vi "aft_LMS_FPGA_Code_Generation.vi"(8 "read coefficient? (F)":bool, 9 "filter name":string, 10 "fixed-point LMS settings":T1, 11 "target item":refnum<vi>) -> (0 "error out":errorcluster, 2 "continue?":bool)   [LabVIEW 2017, in "NI_AdaptiveFilter.lvlib"]
uses:
  <vilib>/addons/Adaptive Filters/NI_AdaptiveFilter.lvlib
  <vilib>/addons/Adaptive Filters/Utilities/AFT Algorithm.ctl
  <vilib>/addons/Adaptive Filters/Utilities/AFT Errors.ctl
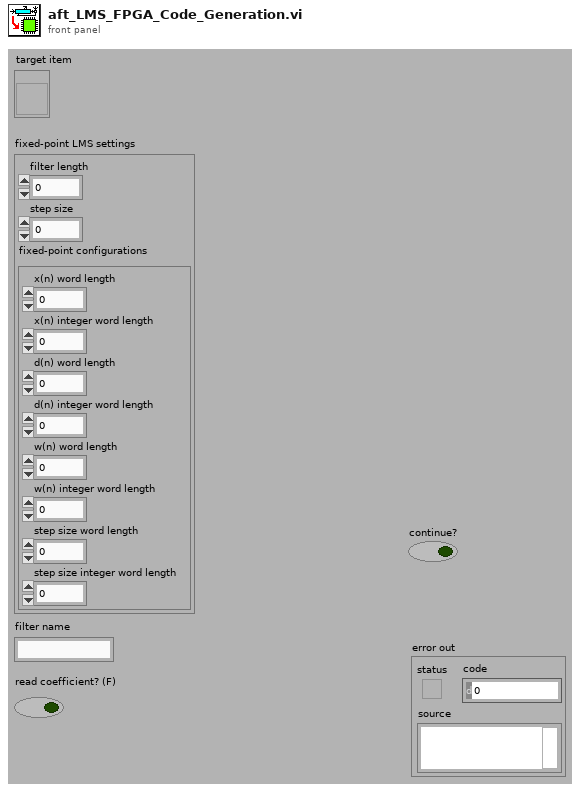
[diagram p1: front panel]
types:
  T1 = cluster{"filter length":i32, "step size":dbl, "fixed-point configurations":cluster{"x(n) word length":i32, "x(n) integer word length":i32, "d(n) word length":i32, "d(n) integer word length":i32, "w(n) word length":i32, "w(n) integer word length":i32, "step size word length":i32, "step size integer word length":i32}}
  T2 = typedef "NI_AdaptiveFilter.lvlib/AFT Errors.ctl" = i32
  T3 = typedef "NI_AdaptiveFilter.lvlib/AFT Algorithm.ctl" = u16
  T4 = cluster{"x(n) word length":i32, "x(n) integer word length":i32, "d(n) word length":i32, "d(n) integer word length":i32, "w(n) word length":i32, "w(n) integer word length":i32, "step size word length":i32, "step size integer word length":i32}
  T5 = cluster{"algorithm":T3, "filter length":i32, "step size":dbl, "fixed-point configurations":cluster{"x(n) word length":i32, "x(n) integer word length":i32, "d(n) word length":i32, "d(n) integer word length":i32, "w(n) word length":i32, "w(n) integer word length":i32, "step size word length":i32, "step size integer word length":i32}}
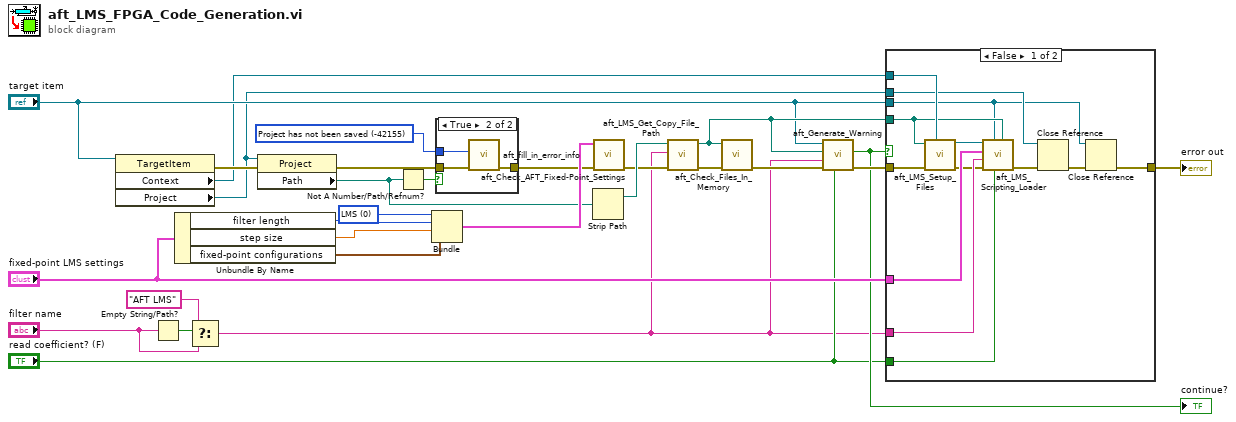
[diagram p0: block diagram]
diagram:
  w12 = T2 -42155 items=["No error"=0, "Sampling interval mismatch"=-42018, "Invalid FPGA target"=-42150, "Invalid filter configurations"=-42151, "LabVIEW FPGA or NI-RIO not installed"=-42152, "Fail to overwrite"=-42153, "File exists in memory"=-42154, "Project has not been saved"=-42155] ("AFT errors")
  w16 = T3 0 items=["LMS"] ("algorithm")
  n1 = property class="TargetItem"(reference="target item") -> (error out=w26:errorcluster, "Context"=w1:refnum<vi>, "Project"=w2:refnum<vi>)  [unwired: 1 in, 1 out]
  n2 = Empty String/Path?(string/path="filter name") -> (empty?=w24:bool)
  n3 = Unbundle By Name("fixed-point LMS settings") -> ("filter length"=w20:i32, "step size"=w19:dbl, "fixed-point configurations"=w18:T4)
  n4 = Select(t="AFT LMS", s=w24, f="filter name") -> (s? t:f=w3:string)
  n5 = property class="Project"(reference=w2, error in=w26) -> (error out=w13:errorcluster, "Path"=w15:path)  [unwired: 1 out]
  n6 = Not A Number/Path/Refnum?(number/path/refnum=w15) -> (NaN/Path/Refnum?=w14:bool)
  n7 = Bundle("algorithm"=w16, "filter length"=w20, "step size"=w19, "fixed-point configurations"=w18) -> (w17:T5)  [unwired: 1 out]
  n8 = case shown="True" w14 {
    tunnel: w13 -> [w29 w32]
    tunnel: [w29 w31] -> w11
    tunnel: w12 -> [_ w30]
    frame False {
    }
    frame True {
      n9 = call <vilib>:"aft_fill_in_error_info.vi"("error in"=w32, "status code"=w30) -> ("error out"=w31:errorcluster)  [unwired: 2 in, 7 out]
    }
  }
  n10 = Strip Path(path=w15) -> (stripped path=w28:path)  [unwired: 1 out]
  n11 = call <vilib>:"aft_Check_AFT_Fixed-Point_Settings.vi"("error in (no error)"=w11, "AFT fixed-point settings"=w17) -> ("error out"=w25:errorcluster)  [unwired: 9 out]
  n12 = call <vilib>:"aft_LMS_Get_Copy_File_Path.vi"("error in"=w25, "filter name"=w3, "destination folder"=w28) -> ("error out"=w27:errorcluster, "destination path"=w5:path)  [unwired: 1 in, 6 out]
  n13 = call <vilib>:"aft_Check_Files_In_Memory.vi"("error in (no error)"=w27, "destination folder"=w5) -> ("error out"=w6:errorcluster)  [unwired: 9 out]
  n14 = call <vilib>:"aft_Generate_Warning.vi"("read coefficient? (F)"="read coefficient? (F)", "error in (no error)"=w6, "memory name"=w3, "destination path"=w5, "target ref"="target item") -> ("error out"=w10:errorcluster, "continue"=w9:bool)  [unwired: 5 in]
  "continue?" <- w9
  n15 = case shown="False" w9 {
    tunnel: w5 -> [w38 _]
    tunnel: w10 -> [w41 w46]
    tunnel: "read coefficient? (F)" -> [w45 _]
    tunnel: w1 -> [w44 _]
    tunnel: w3 -> [w43 _]
    tunnel: "fixed-point LMS settings" -> [w42 _]
    tunnel: "target item" -> [w36 _]
    tunnel: [w33 w46] -> w8
    tunnel: w2 -> [w37 _]
    frame False {
      n16 = call <vilib>:"aft_LMS_Setup_Files.vi"("application reference (local)"=w44, "error in (no error)"=w41, "destination path"=w38) -> ("error out"=w39:errorcluster, "VI"=w40:refnum<vi>)  [unwired: 1 in, 6 out]
      n17 = call <vilib>:"aft_LMS_Scripting_Loader.vi"("destination path"=w38, "read coefficient? (F)"=w45, "TargetItem Refnum"=w36, "error in"=w39, "filter name"=w43, "fixed-point LMS settings"=w42, "VI in"=w40) -> ("error out"=w35:errorcluster)  [unwired: 1 in, 3 out]
      n18 = Close Reference(reference=w37, error in (no error)=w35) -> (error out=w34:errorcluster)
      n19 = Close Reference(reference=w36, error in (no error)=w34) -> (error out=w33:errorcluster)
    }
    frame True {
    }
  }
  "error out" <- w8
